vi "Check Response.vi"(7 "Nest Error":T2, 8 "Error In":errorcluster, 9 "Body":string, 10 "Header":string, 11 "Client Handle":T1) -> (0 "Error Out":errorcluster, 1 "Success?":bool, 2 "Body":string, 3 "Client Handle":T1)   [LabVIEW 2013, in "LMH-Nest.lvlib"]
doc: "Check HTTP response from Nest server. Generate error if response indicates communicaiton failure."
uses:
  LMH-Nest.lvlib
  <vilib>/httpClient/ClientHandle.ctl
  Type Defs/Nest Error.ctl
  <vilib>/httpClient/LabVIEWHTTPClient.lvlib
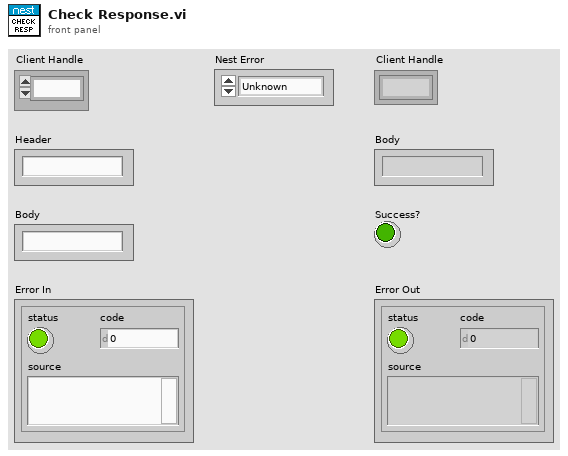
[diagram p1: front panel]
types:
  T1 = typedef "LabVIEWHTTPClient.lvlib/ClientHandle.ctl" = refnum<k1>
  T2 = typedef "LMH-Nest.lvlib/Nest Error.ctl" = enum16{"Unknown", "Auth", "Read", "Invalid Structure Name", "Invalid Device Name", "Set Temp"}
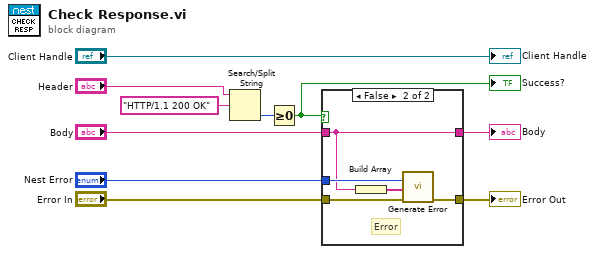
[diagram p0: block diagram]
diagram:
  n1 = Search/Split String(string="Header", search string/char (-)="HTTP/1.1 200 OK") -> (offset of match=w9:i32)  [unwired: 1 in, 2 out]
  n2 = Greater Or Equal To 0?(x=w9) -> (x >= 0?=w7:bool)
  "Success?" <- w7
  n3 = case shown="False" w7 {
    tunnel: "Nest Error" -> [_ w15]
    tunnel: "Body" -> [w11 w13]
    tunnel: "Error In" -> [w12 w17]
    tunnel: [w12 w16] -> w3
    tunnel: [w11 w13] -> w1
    frame True {
      # "Success"
    }
    frame False {
      # "Error"
      n4 = Build Array(w13) -> (w14:string[])
      n5 = call "Generate Error.vi"("Error In"=w17, "Args"=w14, "Nest Error"=w15) -> ("Error Out"=w16:errorcluster)  [unwired: 8 in]
    }
  }
  "Error Out" <- w3
  "Body" <- w1
  "Client Handle" <- "Client Handle"
